vi "old_rqcAlice SPI.Set Att Value.vi"(8 "error in":errorcluster, 10 "Attenuation, dB":fxp<+,7,6>, 11 "Alice FPGA Reference In":refnum<k20>) -> (0 "error out":errorcluster, 3 "Alice FPGA Reference Out":refnum<k20>)   [LabVIEW 2019]
uses:
  Shared/Shared Host Lib/SPI/typedefs/SPI.FPGA Interface.ctl
  Shared/Shared Host Lib/SPI/typedefs/SPI.SubSystem.ctl
  <vilib>/Utility/error.llb/Error Cluster From Error Code.vi
  <vilib>/rvi/errors/niLvFpgaAdjustHostInterfaceError.vi
  <vilib>/rvi/interface/nirviReadWriteControl/nirviReadWriteControl.xnode
  NiFpgaLv.dll
  <vilib>/rvi/interface/Simulation/niFpgaSimulationCallBeginRW.vi
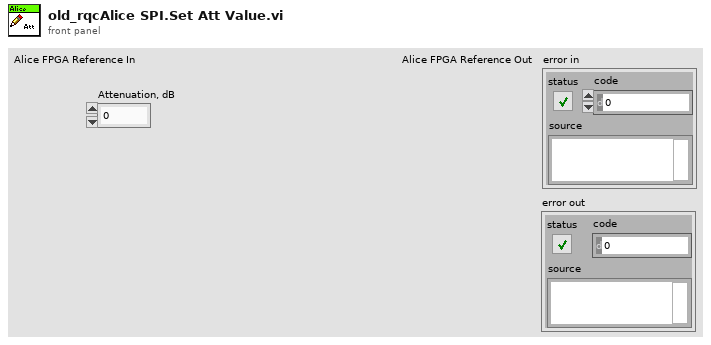
[diagram p1: front panel]
types:
  T1 = typedef "SPI.SubSystem.ctl" = enum8{"N/A", "DelayLine.MSB", "DelayLine.LSB", "Attenuation.dB", "Attenuation.DAC value", "SyncDetector.Offset", "SyncDetector.Comparator", "PM.Value[0]", "PM.Value[1]", "PM.Value[2]", "PM.Value[3]"}
  T2 = typedef "SPI.FPGA Interface.ctl" = refnum<k20>
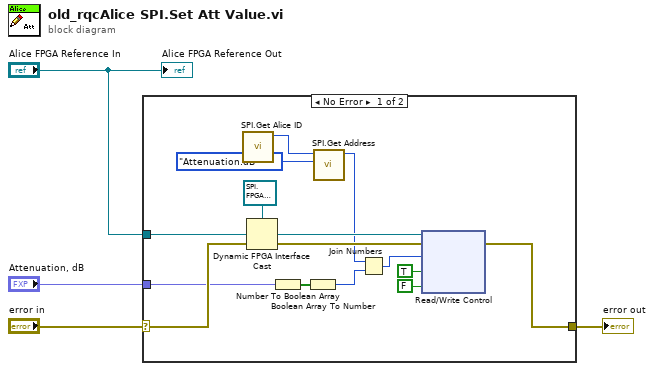
[diagram p0: block diagram]
diagram:
  n1 = case shown="No Error" "error in" {
    selector: "error in" -> [w12 w19]
    tunnel: [w8 w19] -> w3
    tunnel: "Alice FPGA Reference In" -> [w18 _]
    tunnel: "Attenuation, dB" -> [w7 _]
    frame No Error {
      n2 = call "SPI.Get Alice ID.vi"() -> ("Alice.ID"=w11:u8)  [unwired: 11 in]
      n3 = Dynamic FPGA Interface Cast(Session In=T2 refnum ("Type"), Type=w18) -> (Session Out=w13:T2)
      n4 = Number To Boolean Array(number=w7) -> (Boolean array=w6:bool[])
      n5 = Boolean Array To Number(Boolean array=w6) -> (number=w5:u16)
      n6 = call "SPI.Get Address.vi"("SPI.subSystem"=SPI.SubSystem."Attenuation.dB", "ID"=w11) -> ("Address"=w10:u16)  [unwired: 9 in]
      n7 = Join Numbers(hi=w10, lo=w5) -> ((hi.lo)=w14:u32)
      n8 = xnode "Read/Write Control"("FPGA VI Reference In"=w13, "error in"=w12, "SPI.data"=w14, "SPI.write"=TRUE ("reset"), "SPI.write"=FALSE ("reset")) -> ("error out"=w8:errorcluster)  [unwired: 1 out]
    }
    frame Error {
    }
  }
  "error out" <- w3
  "Alice FPGA Reference Out" <- "Alice FPGA Reference In"
